vi "Create Unique File.vi"(8 "error in (no error)":errorcluster, 11 "appended path":path) -> (0 "error out":errorcluster, 3 "Byte Stream File out":refnum<file>)   [LabVIEW 2016, in "BTL_logger.lvlib"]
uses:
  BTL_logger.lvlib
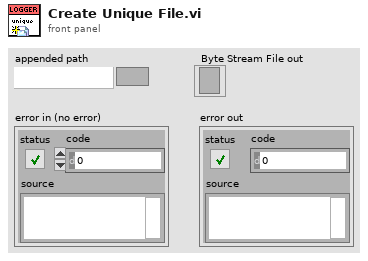
[diagram p1: front panel]
types:
  T1 = enum16{"open", "replace", "create", "open or create", "replace or create", "replace or create with confirmation"}
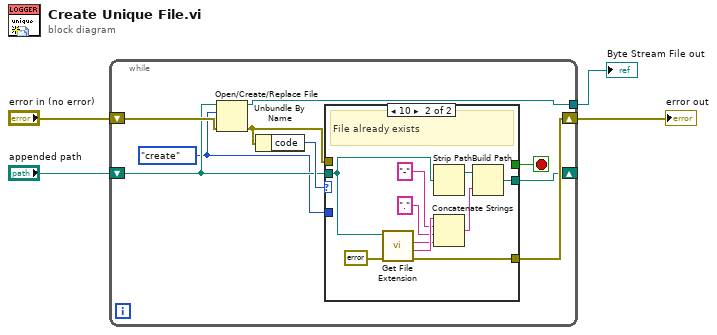
[diagram p0: block diagram]
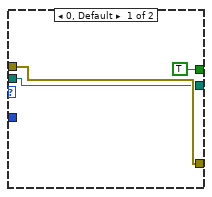
[diagram p2: hidden frame]
diagram:
  n1 = while {
    tunnel: [w5] -> w3
    shift-right: [w11] -> w2
    shift-left: "error in (no error)" -> [w13]
    shift-right: [w6] -> _
    shift-left: "appended path" -> [w9]
    stop <- w7 stop-if-true
    w8 = T1."create" ("operation (0:open)")
    n2 = Open/Create/Replace File(file path (use dialog)=w9, error in=w13, operation (0:open)=w8) -> (refnum out=w5:refnum<file>, error out=w10:errorcluster)  [unwired: 3 in, 1 out]
    n3 = Unbundle By Name(w10) -> ("code"=w12:i32)
    n4 = case shown="10" w12 {
      tunnel: [w16 w22] -> w11
      tunnel: w10 -> [w16 _]
      tunnel: w9 -> [w14 w18]
      tunnel: w8 -> [_ _]
      tunnel: [TRUE _] -> w7
      tunnel: [w14 w19] -> w6
      frame 0, Default {
      }
      frame 10 {
        # "File already exists"
        n5 = call <vilib>:"Get File Extension.vi"("error in (no error)"=errorcluster {"status"=FALSE, "code"=0, "source"=""} ("error in"), "file"=w18) -> ("error out"=w22:errorcluster, "filename without extension"=w25:string, "lowercase file extension"=w21:string)  [unwired: 5 in, 2 out]
        n6 = Strip Path(path=w18) -> (stripped path=w17:path)  [unwired: 1 out]
        n7 = Concatenate Strings(w25, "-" ("string"), "." ("string"), w21) -> (w24:string)
        n8 = Build Path(base path=w17, name or relative path=w24) -> (appended path=w19:path)
      }
    }
  }
  "Byte Stream File out" <- w3
  "error out" <- w2
